vi "Globalmanueel.vi"() -> ()   [LabVIEW 2019]
panel:
  in  "MANUEEL":bool
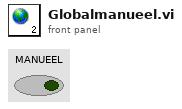
[diagram p1: front panel]
diagram:
